vi "StressDist_long_costEval.vi"(8 "Error In":errorcluster, 10 "Data":variant, 11 "Elements":T1[](array[typedef])) -> (0 "Error Out":errorcluster, 3 "Elements out":T1[](array[typedef]))   [LabVIEW 2016]
uses:
  UserLibraries/AlgoritmoGenetico/TypeDefs/element.ctl
  StressCalculations/point_data.ctl
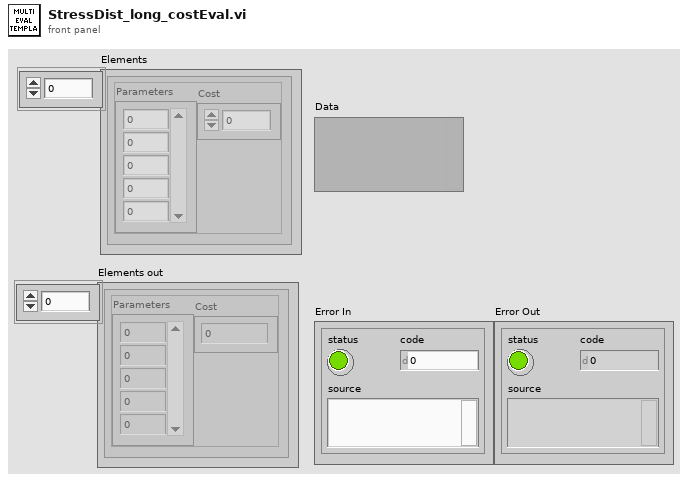
[diagram p1: front panel]
types:
  T1 = typedef "element.ctl" = cluster{"Parameters":dbl[], "Cost":dbl}
  T2 = typedef "point_data.ctl" = cluster{"LongStress":dbl, "CircStress":dbl, "ShearStress":dbl, "Pressure":dbl, "Angle":dbl, "Thickness":dbl, "HoleDiam":dbl}
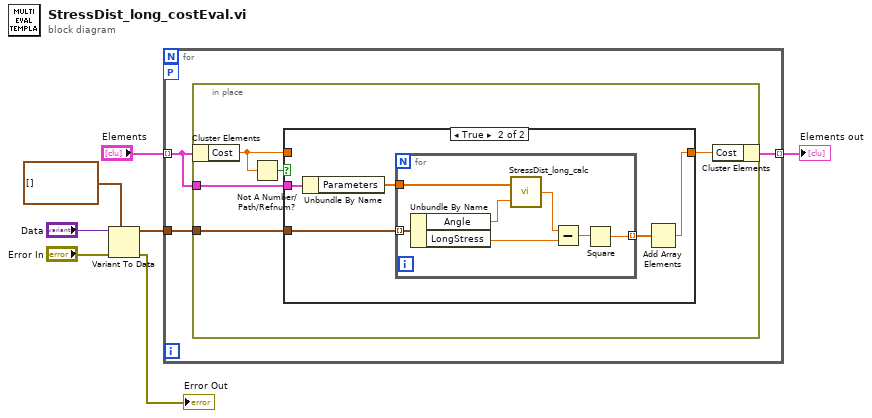
[diagram p0: block diagram]
diagram:
  n1 = Variant To Data(error in="Error In", type=T2[] [] ("Points"), Variant="Data") -> (data=w3:T2[], error out=→"Error Out":errorcluster)
  n2 = for {
    workers-P: _ -> [_]
    tunnel: "Elements" -> [w10] mode=indexing
    tunnel: w3 -> [w9]
    tunnel: [w8] -> w2 mode=indexing
    n3 = in-place {
      in-place-border: w10 -> [w12]
      in-place-border: w9 -> [w11]
      n4 = in-place-cluster #1(w10) -> ("Cost"=w14:dbl)
      n5 = Not A Number/Path/Refnum?(number/path/refnum=w14) -> (NaN/Path/Refnum?=w15:bool)
      n6 = case shown="True" w15 {
        tunnel: w14 -> [w16 _]
        tunnel: [w16 w17] -> w13
        tunnel: w12 -> [_ w21]
        tunnel: w11 -> [_ w19]
        frame False {
        }
        frame True {
          n7 = Unbundle By Name(w21) -> ("Parameters"=w20:dbl[])
          n8 = for {
            tunnel: w20 -> [w23]
            tunnel: w19 -> [w28] mode=indexing
            tunnel: [w24] -> w18 mode=indexing
            n9 = Unbundle By Name(w28) -> ("Angle"=w22:dbl, "LongStress"=w26:dbl)
            n10 = call "StressDist_long_calc.vi"("Angle"=w22, "Parameters"=w23) -> ("Stress"=w27:dbl)
            n11 = Subtract(x=w27, y=w26) -> (x-y=w25:dbl)
            n12 = Square(x=w25) -> (x^2=w24:dbl)
          }
          n13 = Add Array Elements(numeric array=w18) -> (sum=w17:dbl)
        }
      }
      n14 = in-place-cluster #1("Cost"=w13) -> (w8:T1)
    }
  }
  "Elements out" <- w2
